vi "WaveformWork.vi"() -> ()   [LabVIEW 2014]
uses:
  <vilib>/measure/NI_MABase.lvlib
panel:
  in  "frequency":dbl=250.0 format="%#_13g"
  in  "sampling info":cluster{"Fs":dbl, "#s":dbl}={"Fs"=1000.0, "#s"=1000.0}
  out "signal out":waveform(dbl)
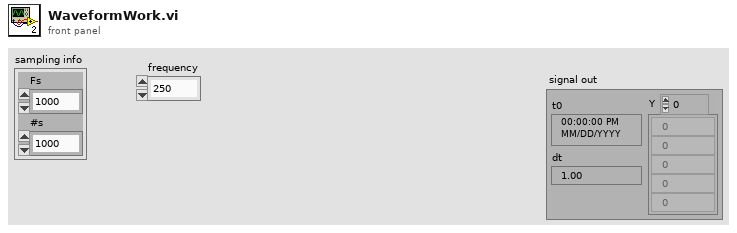
[diagram p1: front panel]
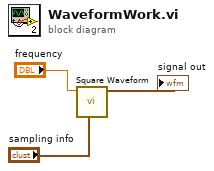
[diagram p0: block diagram]
diagram:
  n1 = call <vilib>:"Square Waveform.vi"("sampling info"="sampling info", "frequency"="frequency") -> ("signal out"=→"signal out":waveform(dbl))  [unwired: 8 in, 1 out]
